vi "FTW-WEB-CreateWebServiceINI.vi"(0 "Output Directory":path, 5 "Service Name":string, 7 "Request Handler Callback Filepaths":path[](array[path]), 9 "Routing Rules":T2(array[cluster]), 11 "error in":errorcluster) -> (4 "INI filepath":path, 15 "error out":errorcluster)   [LabVIEW 2013]
uses:
  <vilib>/AppBuilder/AB_Classes/RESTful/AB_RESTful_HTTPMethodType.ctl
  <vilib>/AppBuilder/Engine/RESTful INI Generator/AB_RESTful_ServiceInfo.ctl
  <vilib>/AppBuilder/Engine/RESTful INI Generator/AB_RESTful_ServiceType.ctl
  <vilib>/AppBuilder/AB_Classes/RESTful/AB_RESTful_ServiceAttribute.ctl
  <vilib>/AppBuilder/AB_Classes/RESTful/AB_RESTful_ServiceAttributeType.ctl
  <vilib>/AppBuilder/AB_Classes/Source/RESTfulVI/Configure_RESTfulVI/AB_RESTful_Configuration.ctl
  <vilib>/AppBuilder/AB_Classes/Source/RESTfulVI/Configure_RESTfulVI/AB_RESTful_VIType.ctl
  <vilib>/AppBuilder/AB_Classes/Source/RESTfulVI/Configure_RESTfulVI/AB_RESTful_OutputType.ctl
  <vilib>/AppBuilder/AB_Classes/Source/RESTfulVI/Configure_RESTfulVI/AB_RESTful_OutputFormat.ctl
  <vilib>/AppBuilder/AB_Classes/RESTful/AB_RESTful_RoutingTemplate.ctl
  <vilib>/AppBuilder/AB_Classes/RESTful/AB_RESTful_RoutingType.ctl
panel:
  # "Inputs"
  # "Outputs"
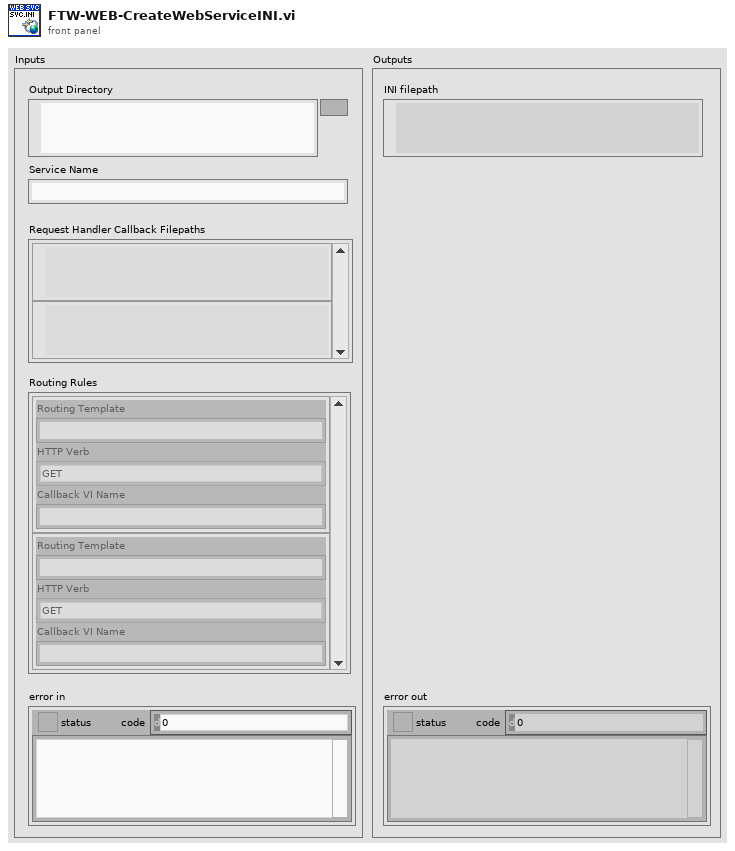
[diagram p1: front panel]
types:
  T1 = typedef "AB_RESTful_HTTPMethodType.ctl" = enum32{"GET", "POST", "PUT", "DELETE"}
  T2 = cluster{"Routing Template":string, "HTTP Verb":T1, "Callback VI Name":string}[]
  T3 = typedef "AB_RESTful_ServiceType.ctl" = enum32{"RESTful", "SOAP"}
  T4 = typedef "AB_RESTful_ServiceInfo.ctl" = cluster{"Service Name":string, "Service Type":T3, "Web Service Library Path":path, "Server List":string[], "Debug":bool, "Service aliases":string[], "defaultStaticDoc":string, "defaultWebMethod":string, "Standalone":bool, "Service attributes":T5[]}
  T5 = typedef "AB_RESTful_ServiceAttribute.ctl" = cluster{"Name":string, "Service Attribute Type":T6, "Value":string}
  T6 = typedef "AB_RESTful_ServiceAttributeType.ctl" = enum32{"String", "Path"}
  T7 = typedef "AB_RESTful_RoutingType.ctl" = enum32{"Method", "Static"}
  T8 = typedef "AB_RESTful_RoutingTemplate.ctl" = cluster{"Template":string, "Routing Type":T7, "HTTP Method Type":T1, "VIName":string, "Default String":string, "Require API key":bool, "Auth permissions":string[], "eng_Static Alias":string}
  T9 = typedef "AB_RESTful_Configuration.ctl" = cluster{"Service VI Type":T10, "Load VI at statup":bool, "Keep VI in memory":bool, "Output type":T11, "Output format":T12, "Use headers":bool, "Buffered":bool, "eng_Load VI by name":bool}
  T10 = typedef "AB_RESTful_VIType.ctl" = enum32{"Web Method", "Auxiliary", "eng_Internal", "eng_Content"}
  T11 = typedef "AB_RESTful_OutputType.ctl" = enum32{"Terminal", "Stream"}
  T12 = typedef "AB_RESTful_OutputFormat.ctl" = enum32{"XML", "Text", "HTML", "JSON"}
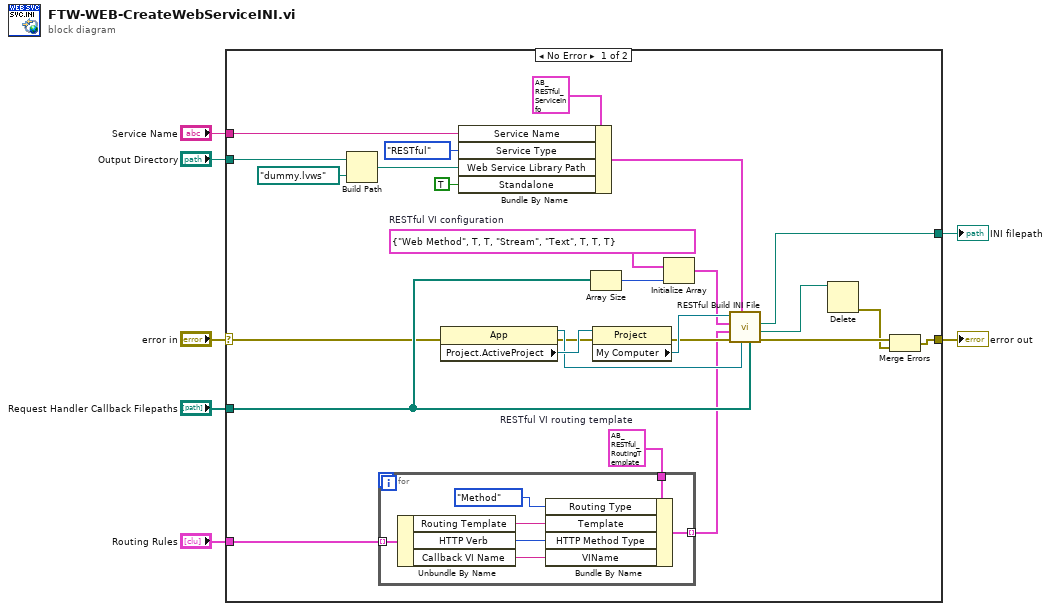
[diagram p0: block diagram]
diagram:
  n1 = case shown="No Error" "error in" {
    selector: "error in" -> [w11 w41]
    tunnel: [w29 _] -> w7
    tunnel: "Output Directory" -> [w10 _]
    tunnel: "Service Name" -> [w25 _]
    tunnel: "Request Handler Callback Filepaths" -> [w20 _]
    tunnel: [w16 w41] -> w3
    tunnel: "Routing Rules" -> [w14 _]
    frame No Error {
      w12 = T8 {"Template"="", "Routing Type"=enum."Static", "HTTP Method Type"=enum."GET", "VIName"="", "Default String"="", "Require API key"=FALSE, "Auth permissions"=[], "eng_Static Alias"=""}  # RESTful VI routing template
      w22 = T9 {"Service VI Type"=enum."Web Method", "Load VI at statup"=TRUE, "Keep VI in memory"=TRUE, "Output type"=enum."Stream", "Output format"=enum."Text", "Use headers"=TRUE, "Buffered"=TRUE, "eng_Load VI by name"=TRUE}  # RESTful VI configuration
      n2 = Build Path(base path=w10, name or relative path=path "dummy.lvws") -> (appended path=w9:path)
      n3 = for {
        tunnel: w14 -> [w38] mode=indexing
        tunnel: [w39] -> w13 mode=indexing
        tunnel: w12 -> [w40]
        n4 = Unbundle By Name(w38) -> ("Routing Template"=w37:string, "HTTP Verb"=w36:T1, "Callback VI Name"=w35:string)
        n5 = Bundle By Name(cluster=w40, "Routing Type"=AB_RESTful_RoutingType."Method", "Template"=w37, "HTTP Method Type"=w36, "VIName"=w35) -> (w39:T8)
      }
      n6 = property class="App"(error in=w11) -> (reference out=w27:refnum<vi>, error out=w23:errorcluster, "Project.ActiveProject"=w31:refnum<vi>)  [unwired: 1 in]
      n7 = Bundle By Name(cluster=T4 {"Service Name"="", "Service Type"=enum."RESTful", "Web Service Library Path"=path "", "Server List"=[], "Debug"=FALSE, "Service aliases"=[], "defaultStaticDoc"="", "defaultWebMethod"="", "Standalone"=FALSE, "Service attributes"=[]} ("RESTful VI service information"), "Service Name"=w25, "Service Type"=AB_RESTful_ServiceType."RESTful", "Web Service Library Path"=w9, "Standalone"=TRUE) -> (w32:T4)
      n8 = Array Size(array=w20) -> (size(s)=w21:i32)
      n9 = property class="Project"(reference=w31, error in=w23) -> (error out=w24:errorcluster, "My Computer"=w30:refnum<vi>)  [unwired: 1 out]
      n10 = Initialize Array(w22, w21) -> (w19:T9[])
      n11 = call <vilib>:"RESTful Build INI File.vi"("relative VI paths"=w20, "buildContext"=w27, "RESTful VI service information"=w32, "error in (no error)"=w24, "Routing Templates"=w13, "VI Configurations"=w19, "target reference"=w30) -> ("error out"=w17:errorcluster, "XML filepath"=w18:path, "INI filepath"=w29:path)  [unwired: 1 in, 1 out]
      n12 = Delete(path (use dialog)=w18) -> (error out=w15:errorcluster)  [unwired: 4 in, 2 out]
      n13 = Merge Errors(w17, w15) -> (w16:errorcluster)
    }
    frame Error {
    }
  }
  "error out" <- w3
  "INI filepath" <- w7
